vi "StellarNet Set Parameters.vi"(6 "Temp  Compensation":bool, 7 "Digitizer Clock Rate Setting":i32=3 min=1 max=3, 8 "error in (no error)":errorcluster, 9 "Optical Smoothing Level":i32 min=0 max=4 step=1, 10 "Number of Scans to Average":i32=1 min=1 max=10000 step=1, 11 "Integration Time (ms)":i32=80 caption="Inter scan delay ms") -> (0 "error out":errorcluster)   [LabVIEW 2023]
uses:
  StellarNet Globals.vi
  C:/Program Files/StellarNet/SpectraWiz/Swdll.dll
panel:
  # "Parameters to set:"
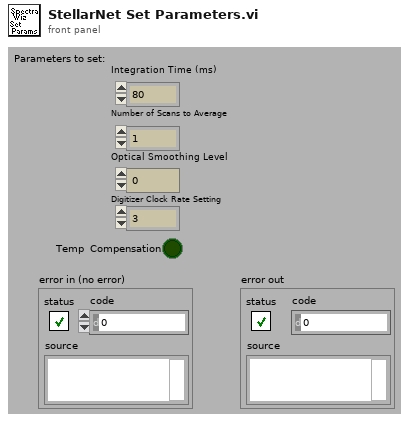
[diagram p1: front panel]
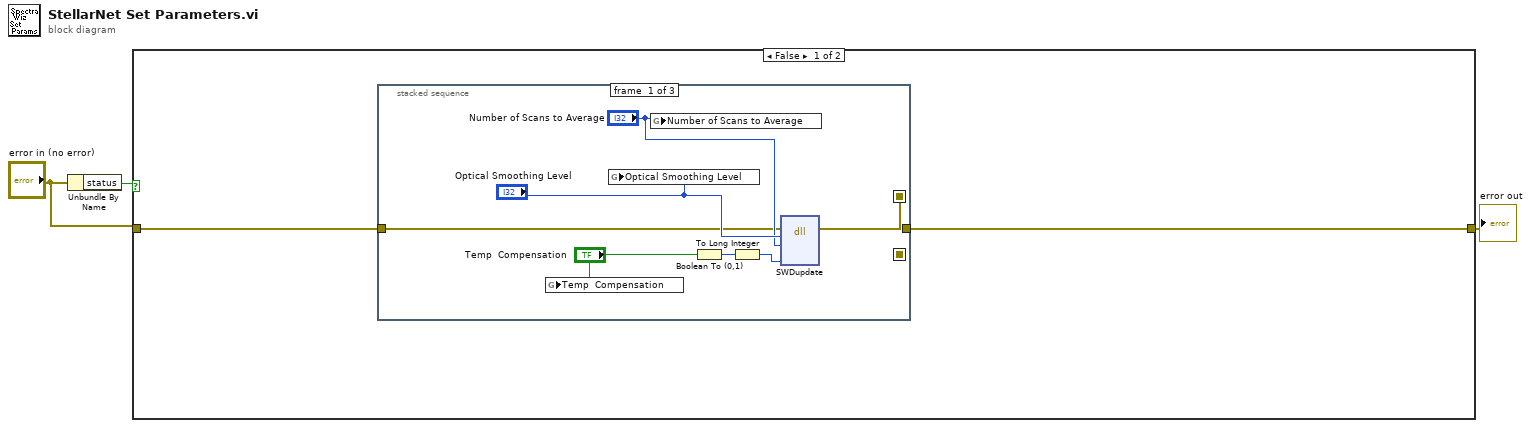
[diagram p0: block diagram]
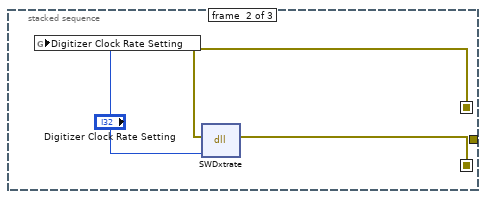
[diagram p2: hidden frame]
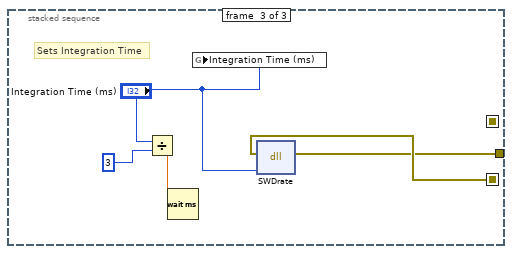
[diagram p3: hidden frame]
diagram:
  n1 = Unbundle By Name("error in (no error)") -> ("status"=w3:bool)
  n2 = case shown="False" w3 {
    tunnel: "error in (no error)" -> [w5 w20]
    tunnel: [w4 w20] -> w1
    frame False {
      n3 = stacked-sequence {
        seq-local: [w6 _ _] -> [_ w13 _]
        seq-local: [_ w12 _] -> [_ _ w19]
        tunnel: w5 -> [w6 _ _]
        tunnel: [_ _ w18] -> w4
        frame #0 {
          n4 = global write "StellarNet Globals.vi" "Temp  Compensation"("Temp  Compensation") -> ()
          n5 = global write "StellarNet Globals.vi" "Optical Smoothing Level"("Optical Smoothing Level") -> ()
          n6 = global write "StellarNet Globals.vi" "Number of Scans to Average"("Number of Scans to Average") -> ()
          n7 = Boolean To (0,1)(Boolean="Temp  Compensation") -> (0, 1=w7:i16)
          n8 = To Long Integer(number=w7) -> (32bit integer=w11:i32)
          n9 = dll-call lib="C:/Program Files/StellarNet/SpectraWiz/Swdll.dll" fn="SWDupdate"(error in=w6, "ScansTo Avg"="Number of Scans to Average", "Xsmooth"="Optical Smoothing Level", "TempComp"=w11) -> ()  [unwired: 6 in, 2 out]
        }
        frame #1 {
          n10 = global write "StellarNet Globals.vi" "Digitizer Clock Rate Setting"("Digitizer Clock Rate Setting") -> ()
          n11 = dll-call lib="C:/Program Files/StellarNet/SpectraWiz/Swdll.dll" fn="SWDxtrate" label="xtrate"(error in=w13, "xtrate"="Digitizer Clock Rate Setting") -> (error out=w12:errorcluster)  [unwired: 4 in, 1 out]
        }
        frame #2 {
          # "Sets Integration Time"
          n12 = Divide(x="Integration Time (ms)", y=3) -> (x/y=w15:dbl)
          n13 = Wait (ms)(milliseconds to wait=w15) -> ()  [unwired: 1 out]
          n14 = global write "StellarNet Globals.vi" "Integration Time (ms)"("Integration Time (ms)") -> ()
          n15 = dll-call lib="C:/Program Files/StellarNet/SpectraWiz/Swdll.dll" fn="SWDrate"(error in=w19, "dsf"="Integration Time (ms)") -> (error out=w18:errorcluster)  [unwired: 4 in, 1 out]
        }
      }
    }
    frame True {
    }
  }
  "error out" <- w1
